vi "Save Parameter.vi"(8 "error in (no error)":errorcluster caption="错误输入（无错误）", 11 "Parameter In":T1) -> (0 "error out":errorcluster caption="错误输出")   [LabVIEW 2023]
uses:
  Ctl/Global Parameter.ctl
  <vilib>/Utility/xml.llb/Write to XML File(string).vi
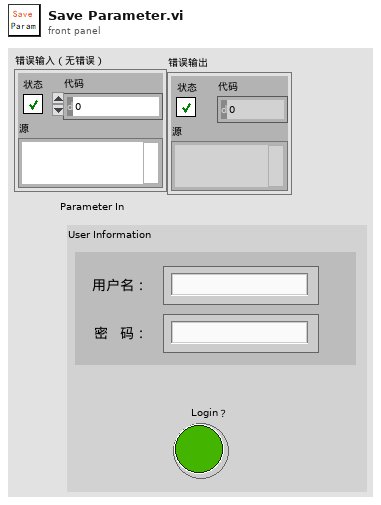
[diagram p1: front panel]
types:
  T1 = typedef "Global Parameter.ctl" = cluster{"User Information":cluster{"用户名：":string, "密   码：":string}, "Login？":bool}
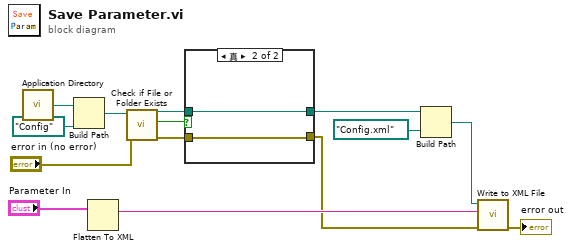
[diagram p0: block diagram]
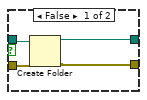
[diagram p2: hidden frame]
diagram:
  n1 = call <vilib>:"Application Directory.vi"() -> ("Application Directory"=w12:path)
  n2 = Build Path(base path=w12, name or relative path=path "Config" ("名称或相对路径")) -> (appended path=w10:path)
  n3 = Flatten To XML(6:"Parameter In") -> (2:w13:string)
  n4 = call <vilib>:"Check if File or Folder Exists.vi"("error in (no error)"="error in (no error)", "path"=w10) -> ("error out"=w7:errorcluster, "file or folder exists?"=w9:bool, "dup path"=w8:path)  [unwired: 7 in]
  n5 = case shown="真" w9 {
    tunnel: w8 -> [w18 w20]
    tunnel: w7 -> [w17 w19]
    tunnel: [w16 w19] -> w2
    tunnel: [w15 w20] -> w6
    frame False {
      n6 = Create Folder(path (use dialog)=w18, error in=w17) -> (created path=w15:path, error out=w16:errorcluster)  [unwired: 1 in, 1 out]
    }
    frame True {
    }
  }
  n7 = Build Path(base path=w6, name or relative path=path "Config.xml" ("名称或相对路径")) -> (appended path=w4:path)
  n8 = call-poly <vilib>:"Write to XML File.vi"("error in (no error)"=w2, "XML Input"=w13, "XML File Path"=w4) -> ("error out"=→"error out":errorcluster)  [unwired: 6 in, 2 out]
